vi "Set Data Ready Call Back.vi"(8 "error in (no error)":errorcluster, 10 "datacallback":cluster{}, 11 "ppara":u32) -> (0 "error out":errorcluster, 3 "ppara out":u32)   [LabVIEW 2021, in "vmmsolib.lvlib"]
doc: "DLL_API void WINAPI SetDataReadyCallBack(void* ppara, DataReadyCallBack datacallback);"
uses:
  vmmsolib.lvlib
  vmmso.dll
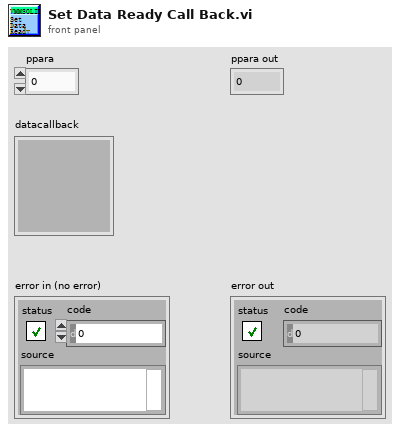
[diagram p1: front panel]
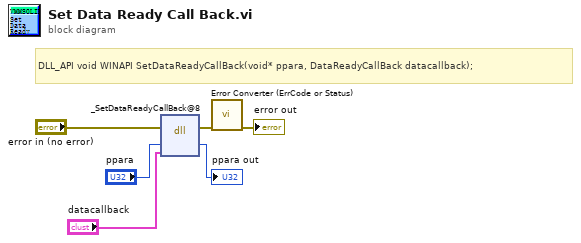
[diagram p0: block diagram]
diagram:
  # "DLL_API void WINAPI SetDataReadyCallBack(void* ppara, DataReadyCallBack datacallback);"
  n1 = dll-call lib="D:/VmMsoSDK/demo-Labview/2021/vmmsolib/vmmso.*" fn="_SetDataReadyCallBack@8"(error in="error in (no error)", "ppara"="ppara", "datacallback"="datacallback") -> (error out=w2:errorcluster, "ppara"=→"ppara out":u32)  [unwired: 4 in, 1 out]
  n2 = call "Error Converter (ErrCode or Status).vi"("error in (no error)"=w2) -> ("error out"=→"error out":errorcluster)  [unwired: 10 in]
